vi "Update Check-out Details.vi"(0 "Rooms Manager Model in":refnum<class "Rooms Manager Model.lvclass">, 5 "Bill Summary":string, 11 "error in (no error)":errorcluster) -> (4 "Rooms Manager Model out":refnum<class "Rooms Manager Model.lvclass">, 15 "error out":errorcluster)   [LabVIEW 2023, in "Rooms Manager Model.lvlib" / "Rooms Manager Model.lvclass"]
uses:
  Rooms Manager Model.lvclass
  Rooms Manager Model.lvclass/Rooms Manager Model.ctl
  Guest Manager Model/Guest Manager Model Messages/Update Guest Name Msg/Update Guest Name Msg.lvclass/Update Guest Name Msg.ctl
  <vilib>/ActorFramework/Message Enqueuer/Message Enqueuer.lvclass/Message Enqueuer.ctl
  <vilib>/ActorFramework/Message Enqueuer/Enqueue.vi
  Guest Manager Model/Guest Manager Model Messages/Update Guest Name Msg/Update Guest Name Msg.lvclass
  C:/Program Files/National Instruments/LabVIEW 2023/vi.lib/ActorFramework/Message/Message.lvclass
  <vilib>/ActorFramework/Message Priority Queue/Priority Enqueue.vi
  Guest Manager Model/Guest Manager Model Messages/Update Check-out Details Msg/Update Check-out Details Msg.lvclass
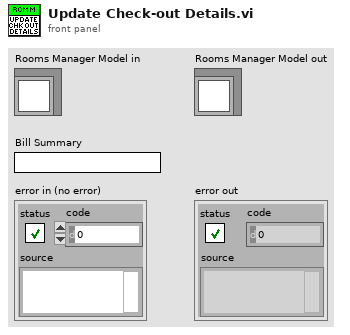
[diagram p1: front panel]
types:
  T1 = typedef "Central Data Manager.lvlib/Central Data Manager.lvclass/Room Details.ctl" = cluster{"Room No":string, "Room Size":string, "Room Occupancy Status":T2, "Guest Details":T3, "Occupancy Count (Adult)":u32, "Occupancy Count (Children)":u32, "Check-in Time":timestamp, "Check-out Time":timestamp}
  T2 = typedef "Central Data Manager.lvlib/Central Data Manager.lvclass/Room Occupancy Status.ctl" = enum16{"Not Occupied", "Occupied", "Under Maintainance", "Not Servicable"}
  T3 = typedef "Central Data Manager.lvlib/Central Data Manager.lvclass/Guest Details.ctl" = cluster{"Contact Number":string, "Primary Guest Name":string}
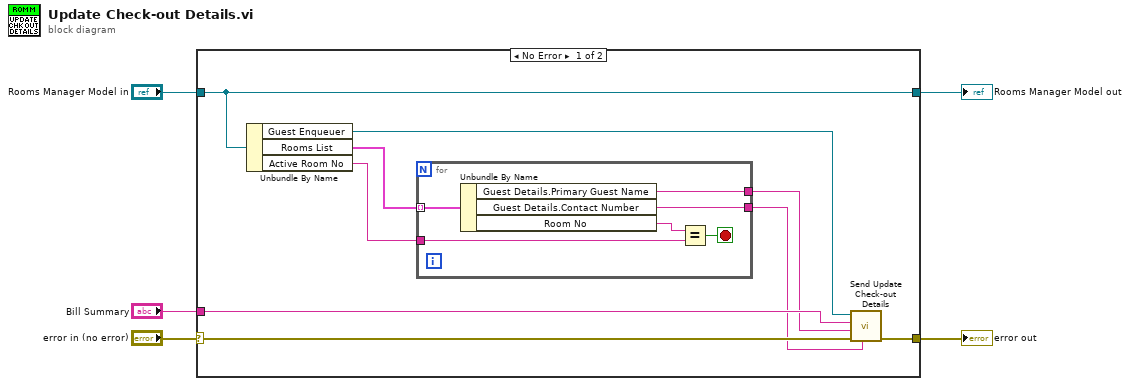
[diagram p0: block diagram]
diagram:
  n1 = case shown="No Error" "error in (no error)" {
    selector: "error in (no error)" -> [w14 w22]
    tunnel: [w13 w22] -> w4
    tunnel: [w12 w21] -> w2
    tunnel: "Rooms Manager Model in" -> [w12 w21]
    tunnel: "Bill Summary" -> [w10 _]
    frame No Error {
      n2 = Unbundle By Name(w12) -> ("Guest Enqueuer"=w11:refnum<class "Message Enqueuer.lvclass">, "Rooms List"=w9:T1[], "Active Room No"=w8:string)
      n3 = for {
        tunnel: w9 -> [w20] mode=indexing
        tunnel: w8 -> [w18]
        tunnel: [w16] -> w7
        tunnel: [w15] -> w6
        stop <- w17 stop-if-true
        n4 = Unbundle By Name(w20) -> ("Guest Details.Primary Guest Name"=w16:string, "Guest Details.Contact Number"=w15:string, "Room No"=w19:string)
        n5 = Equal?(x=w19, y=w18) -> (x = y?=w17:bool)
      }
      n6 = call "Send Update Check-out Details.vi"("Guest Contact Number"=w6, "error in (no error)"=w14, "Primary Guest Name"=w7, "Bill Summary"=w10, "Message Enqueuer"=w11) -> ("error out"=w13:errorcluster)  [unwired: 5 in, 1 out]
    }
    frame Error {
    }
  }
  "error out" <- w4
  "Rooms Manager Model out" <- w2
